vi "Pulse_length.vi"(8 "Sample rate":dbl, 9 "Position in time":dbl[](array[numeric]), 10 "Amplitudes":dbl[](array[numeric]), 11 "Signal":waveform(dbl)) -> (0 "Length of pulses":dbl[](array[numeric]))   [LabVIEW 2020]
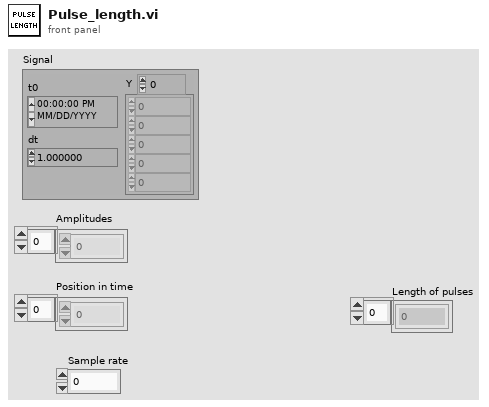
[diagram p1: front panel]
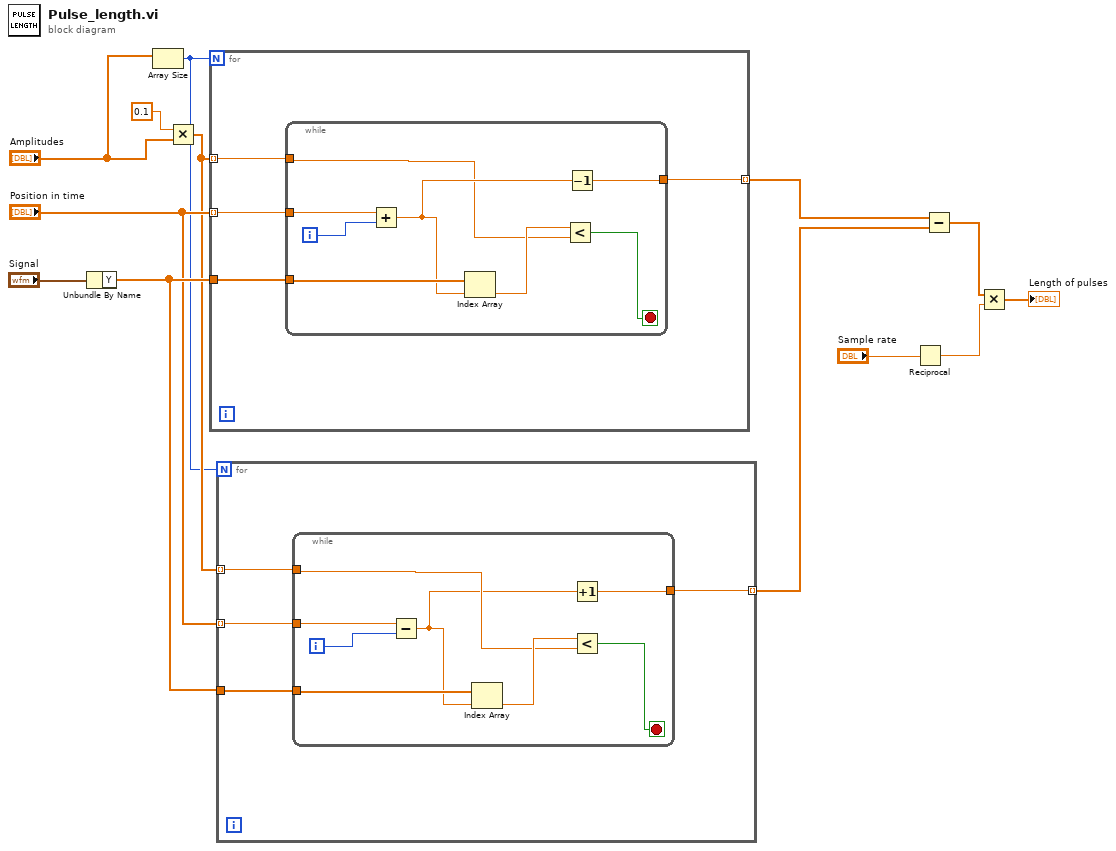
[diagram p0: block diagram]
diagram:
  n1 = Unbundle By Name("Signal") -> ("Y"=w10:dbl[])
  n2 = Array Size(array="Amplitudes") -> (size(s)=w7:i32)
  n3 = Multiply(x=0.1, y="Amplitudes") -> (x*y=w8:dbl[])
  n4 = for {
    N: w7 -> [_]
    tunnel: w10 -> [w17]
    tunnel: w8 -> [w16] mode=indexing
    tunnel: "Position in time" -> [w15] mode=indexing
    tunnel: [w14] -> w2 mode=indexing
    n5 = while {
      tunnel: w17 -> [w23]
      tunnel: w16 -> [w18]
      tunnel: w15 -> [w25]
      tunnel: [w19] -> w14
      i -> [w24]
      stop <- w21 stop-if-true
      n6 = Add(x=w25, y=w24) -> (x+y=w20:dbl)
      n7 = Index Array(array=w23, index=w20) -> (element=w22:dbl)
      n8 = Less?(x=w22, y=w18) -> (x < y?=w21:bool)
      n9 = Decrement(x=w20) -> (x-1=w19:dbl)
    }
  }
  n10 = for {
    N: w7 -> [_]
    tunnel: w10 -> [w29]
    tunnel: w8 -> [w28] mode=indexing
    tunnel: "Position in time" -> [w27] mode=indexing
    tunnel: [w26] -> w1 mode=indexing
    n11 = while {
      tunnel: w29 -> [w37]
      tunnel: w28 -> [w34]
      tunnel: w27 -> [w33]
      tunnel: [w30] -> w26
      i -> [w32]
      stop <- w35 stop-if-true
      n12 = Subtract(x=w33, y=w32) -> (x-y=w31:dbl)
      n13 = Index Array(array=w37, index=w31) -> (element=w36:dbl)
      n14 = Increment(x=w31) -> (x+1=w30:dbl)
      n15 = Less?(x=w36, y=w34) -> (x < y?=w35:bool)
    }
  }
  n16 = Reciprocal(x="Sample rate") -> (1/x=w5:dbl)
  n17 = Subtract(x=w2, y=w1) -> (x-y=w4:dbl[])
  n18 = Multiply(x=w4, y=w5) -> (x*y=→"Length of pulses":dbl[])
